vi "Material-CallArray-Delete0s.vi"(0 "CalData Line 3":dbl[](array[numeric])) -> (1 "array w/ subset deleted":dbl[](array[numeric]))   [LabVIEW 2013, in "Material-RunTest.lvclass"]
uses:
  Material-RunTest.lvclass
  <userlib>/_OpenG.lib/array/array.llb/Search 1D Array (DBL)__ogtk.vi
  <userlib>/_OpenG.lib/array/array.llb/Delete Elements from 1D Array (DBL)__ogtk.vi
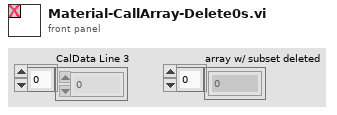
[diagram p1: front panel]
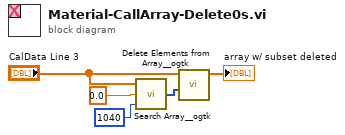
[diagram p0: block diagram]
diagram:
  n1 = call-poly <userlib>:"Search Array__ogtk.vi"("Array"="CalData Line 3", "Element Data"=0.0, "Start Index (0)"=1040) -> ("Indices of Elements"=w3:i32[])  [unwired: 6 in]
  n2 = call-poly <userlib>:"Delete Elements from Array__ogtk.vi"("indices"=w3, "array"="CalData Line 3") -> ("array w/ subset deleted"=→"array w/ subset deleted":dbl[])  [unwired: 8 in, 1 out]
